vi "PicoScope6000ExampleBlockMultiUnit.vi"() -> ()   [LabVIEW 2010]
uses:
  shared/PicoBuffers.ctl
  shared/Buffer and Transfer Settings.ctl
  shared/Acquisition Settings.ctl
  PicoScope6000Lib/PicoScope6000AnalogChannelSettings.ctl
panel:
  out "Overflow":i16[](array[numeric]) format="%04b"
  in  "Trigger Settings":T1={"Trigger Enabled"=FALSE, "Trigger Source"=enum."Channel A", "Trigger Threshold (Volts)"=0.0, "Trigger Direction"=2, "Trigger Delay (samples)"=0, "Auto Trigger Time (ms)"=1000} {"Trigger Direction" items=["Rising"=2, "Falling"=3]}
  in  "Scope Index":i32
  out "Scope \"N\"":cluster{i32, sgl, "Data":dbl[]}[](graph)
  in  "Channel B Settings":T2={"Enabled"=FALSE, "Coupling"=1, "Range"=6, "Analogue Offset"=0.0, "Bandwidth"=0} {"Bandwidth" items=["Full", "20 MHz"]; "Range" items=["10 mV", "20 mV", "50 mV", "100 mV", "200 mV", "500 mV", "1 V", "2 V", "5 V", "10 V", "20 V", "50 V ", "100 V"]; "Coupling" items=["AC", "DC 1 MOhm", "DC 50 Ohm"]}
  out "Device Info":T3(array[cluster])
  out "Properties Panel":T4(array[cluster]) {"Max Total Capture Time Available (sec)" format="%.3p"; "Sample Frequency" format="%.3p"; "Sample Internal" format="%.3p"; "Max Samples Available" format="%.3p"; "Total Capture Time (sec)" format="%.3p"}
  in  "Channel A Settings":T2={"Enabled"=TRUE, "Coupling"=1, "Range"=6, "Analogue Offset"=0.0, "Bandwidth"=0} {"Bandwidth" items=["Full", "20 MHz"]; "Range" items=["10 mV", "20 mV", "50 mV", "100 mV", "200 mV", "500 mV", "1 V", "2 V", "5 V", "10 V", "20 V", "50 V ", "100 V"]; "Coupling" items=["AC", "DC 1 MOhm", "DC 50 Ohm"]}
  in  "Acquisition Settings":T5={"preTriggerSamples"=0, "postTriggerSamples"=5000000, "timebase"=5} {"postTriggerSamples" format="%_6p"; "preTriggerSamples" format="%_6p"}
  in  "Buffer and Transfer Settings":T6={"startIndex"=0, "Samples"=5000000, "Down Sample Ratio"=1, "Down-Sample Mode"=0} {"Down-Sample Mode" items=["RAW none"=2147483648, "None"=0, "Aggregate"=1, "Decimate"=2, "Average"=4]; "Down Sample Ratio" step=1; "Samples" format="%_6p"}
  in  "stop":bool
  in  "Apply Settings":bool
  in  "Serial Number":string[](array[string])
  in  "Use Serial Number":bool
  in  "error in (no error)":errorcluster
  # "Bit 0 = ChA"
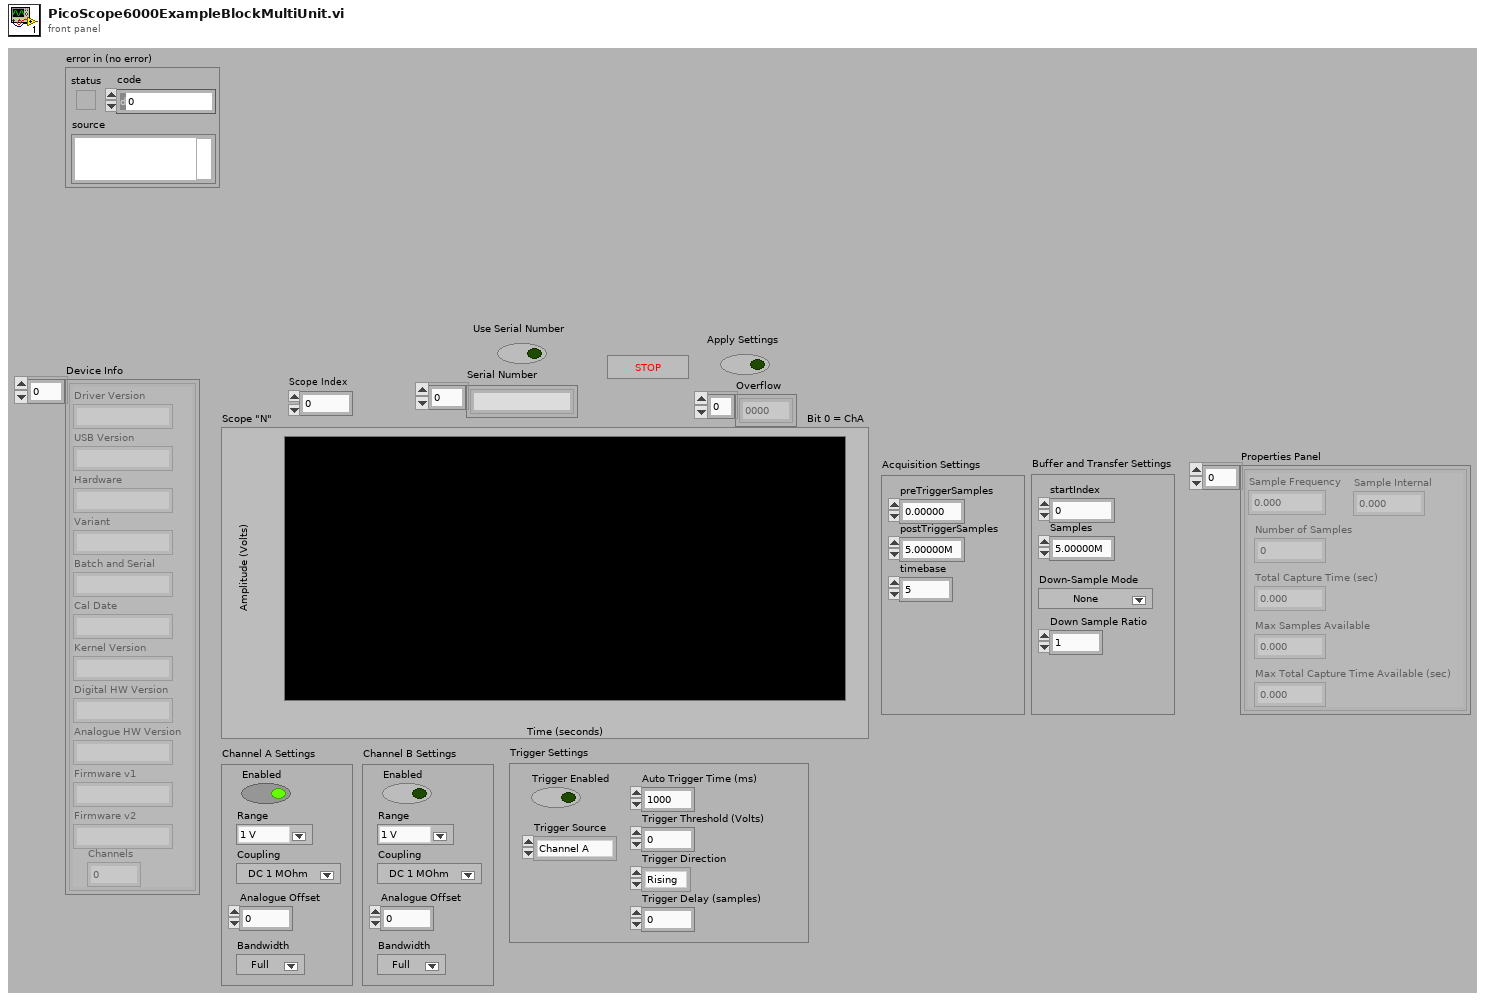
[diagram p1: front panel]
types:
  T1 = cluster{"Trigger Enabled":bool, "Trigger Source":enum32{"Channel A", "Channel B", "Channel C", "Channel D", "External", "Aux."}, "Trigger Threshold (Volts)":dbl, "Trigger Direction":u16, "Trigger Delay (samples)":u32, "Auto Trigger Time (ms)":i16}
  T2 = typedef "PicoScope6000AnalogChannelSettings.ctl" = cluster{"Enabled":bool, "Coupling":u32, "Range":u32, "Analogue Offset":sgl, "Bandwidth":u32}
  T3 = cluster{"Driver Version":string, "USB Version":string, "Hardware":string, "Variant":string, "Batch and Serial":string, "Cal Date":string, "Kernel Version":string, "Digital HW Version":string, "Analogue HW Version":string, "Firmware v1":string, "Firmware v2":string, "Channels":i16}[]
  T4 = cluster{"Sample Frequency":sgl, "Sample Internal":sgl, "maxSamples":u32, "Number of Samples":u32, "Total Capture Time (sec) ":sgl, "Max Total Capture Time Available (sec)":sgl}[]
  T5 = typedef "Acquisition Settings.ctl" = cluster{"preTriggerSamples":u64, "postTriggerSamples":u64, "timebase":u32}
  T6 = typedef "Buffer and Transfer Settings.ctl" = cluster{"startIndex":u64, "Samples":u64, "Down Sample Ratio":u64, "Down-Sample Mode":u32}
  T7 = typedef "PicoBuffers.ctl" = cluster{"Max Buffer Pointers":u64[][][], "Min Buffer Pointers":u64[][][], "StreamingDataInfo":cluster{"Channel":u32, "Down-Sample Mode":u32, "PICO_DATA_TYPE":enum32{"PICO_INT8_T", "PICO_INT16_T", "PICO_INT32_T", "PICO_UINT32_T", "PICO_INT64_T", ""}, "Samples":i32, "bufferIndex":u64, "startIndex":i32, "overflow":i16}[][]}
  T8 = cluster{"Driver Version":string, "USB Version":string, "Hardware":string, "Variant":string, "Batch and Serial":string, "Cal Date":string, "Kernel Version":string, "Digital HW Version":string, "Analogue HW Version":string, "Firmware v1":string, "Firmware v2":string, "Channels":i16}
  T9 = cluster{"Sample Frequency":sgl, "Sample Internal":sgl, "maxSamples":u32, "Number of Samples":u32, "Total Capture Time (sec) ":sgl, "Max Total Capture Time Available (sec)":sgl}
  T10 = cluster{"Channel A Buffer":i16[], "Channel B Buffer":i16[], "Channel C Buffer":i16[], "Channel D Buffer":i16[], "Channel E Buffer":i16[], "Channel F Buffer":i16[], "Channel G Buffer":i16[], "Channel H Buffer":i16[], "Port 0 Buffer":i16[], "Port 1 Buffer":i16[]}[]
  T11 = cluster{"Channel A Buffer":i16[], "Channel B Buffer":i16[], "Channel C Buffer":i16[], "Channel D Buffer":i16[], "Channel E Buffer":i16[], "Channel F Buffer":i16[], "Channel G Buffer":i16[], "Channel H Buffer":i16[], "Port 0 Buffer":i16[], "Port 1 Buffer":i16[]}
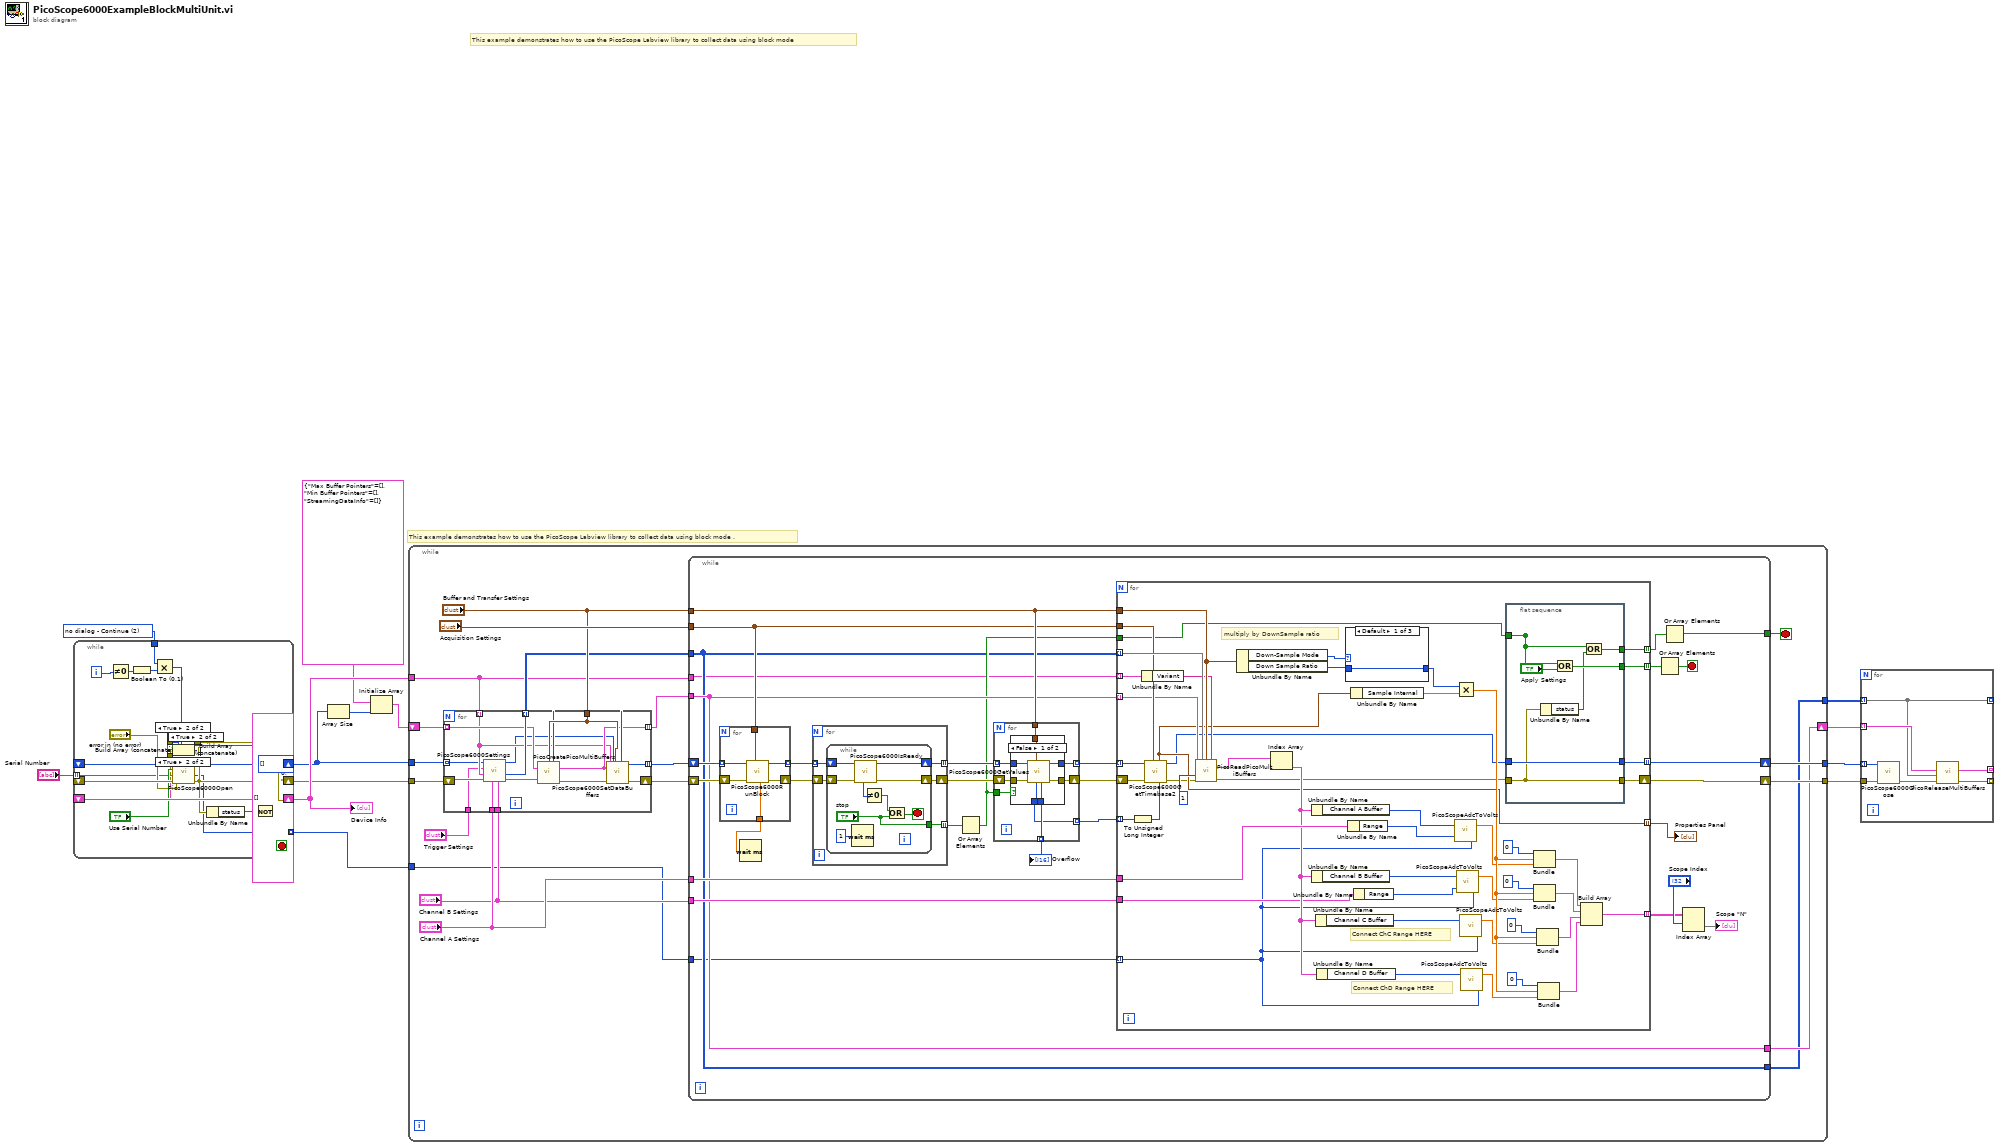
[diagram p0: block diagram]
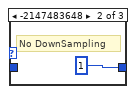
[diagram p5: hidden frame]
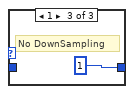
[diagram p6: hidden frame]
diagram:
  w16 = u16 2 items=["Dialog On Error", "no dialog - CloseUnit and Stop", "no dialog - Continue", "no dialog - Stop"] ("Mode")
  # "This example demonstrates how to use the PicoScope Labview library to collect data using block mode ."
  # "This example demonstrates how to use the PicoScope Labview library to collect data using block mode"
  n1 = while {
    tunnel: w16 -> [w30]
    tunnel: "Serial Number" -> [w27] mode=indexing
    tunnel: [w26] -> w8 mode=indexing
    shift-right: [w21] -> w14
    shift-left: errorcluster {"status"=FALSE, "code"=0, "source"=""} ("error out") -> [w22]
    shift-right: [w19] -> w10
    shift-left: i16[] [] ("Array") -> [w20]
    shift-right: [w17] -> w15
    shift-left: T3 [] ("Array") -> [w18]
    i -> [w31]
    stop <- w23 stop-if-true
    n2 = Not Equal To 0?(x=w31) -> (x != 0?=w33:bool)
    n3 = Boolean To (0,1)(Boolean=w33) -> (0, 1=w32:i16)
    n4 = Multiply(x=w30, y=w32) -> (x*y=w29:u16)
    n5 = call "PicoScope6000Open.vi"("Mode"=w29, "error in (no error)"="error in (no error)", "Serial Number"=w27, "Use Serial Number"="Use Serial Number") -> ("error out"=w28:errorcluster, "Max Adc value"=w26:i16, "handle"=w25:i16, "Device Info"=w34:T8)  [unwired: 3 in, 1 out]
    n6 = Unbundle By Name(w28) -> ("status"=w23:bool)
    n7 = Not(x=w23) -> (.not. x?=w24:bool)
    n8 = case shown="True" w24 {
      tunnel: w18 -> [w37 w39]
      tunnel: w34 -> [_ w38]
      tunnel: [w37 w40] -> w17
      frame False {
      }
      frame True {
        n9 = Build Array (concatenate)(w39, w38) -> (w40:T3)
      }
    }
    n10 = case shown="True" w24 {
      tunnel: w20 -> [w41 w43]
      tunnel: w25 -> [_ w42]
      tunnel: [w41 w44] -> w19
      frame False {
      }
      frame True {
        n11 = Build Array (concatenate)(w43, w42) -> (w44:i16[])
      }
    }
    n12 = case shown="True" w24 {
      tunnel: w22 -> [w45 _]
      tunnel: w28 -> [_ w46]
      tunnel: [w45 w46] -> w21
      frame False {
      }
      frame True {
      }
    }
  }
  "Device Info" <- w15
  n13 = Array Size(array=w10) -> (size(s)=w12:i32)
  n14 = Initialize Array(T7 {"Max Buffer Pointers"=[], "Min Buffer Pointers"=[], "StreamingDataInfo"=[]} ("Data Pointers"), w12) -> (w9:T7[])
  n15 = while {
    tunnel: w14 -> [w50]
    tunnel: [w49] -> w5
    tunnel: w15 -> [w55]
    tunnel: w10 -> [w51]
    tunnel: [w64] -> w7
    tunnel: [w62] -> w4
    shift-right: [w52] -> w6
    shift-left: w9 -> [w53]
    tunnel: w8 -> [w48]
    stop <- w63 stop-if-true
    n16 = for {
      tunnel: [w79] -> w60 mode=indexing
      tunnel: "Channel A Settings" -> [w77]
      tunnel: "Buffer and Transfer Settings" -> [w76]
      tunnel: [w75] -> w57 mode=indexing
      tunnel: w55 -> [w71] mode=indexing
      tunnel: "Channel B Settings" -> [w73]
      tunnel: w51 -> [w69] mode=indexing
      shift-right: [w80] -> w61
      shift-left: w50 -> [w70]
      tunnel: w53 -> [w72] mode=indexing
      tunnel: [w74] -> w56 mode=indexing
      tunnel: "Trigger Settings" -> [w66]
      n17 = call "PicoScope6000Settings.vi"("Channel B Settings"=w73, "Channel A Settings"=w77, "error in"=w70, "Device Info"=w71, "Trigger Settings"=w66, "handle in"=w69) -> ("error out"=w68:errorcluster, "Enabled array"=w75:i16[], "handle out"=w67:i16)  [unwired: 3 in]
      n18 = call "PicoCreatePicoMultiBuffers.vi"("Buffer and Transfer Settings"=w76, "enabled array"=w75, "Data Pointers In"=w72, "error in (no error)"=w68) -> ("Data Pointers"=w74:T7, "error out"=w78:errorcluster)  [unwired: 10 in]
      n19 = call "PicoScope6000SetDataBuffers.vi"("enabled array"=w75, "Buffer and Transfer Settings"=w76, "error in (no error)"=w78, "Device Info"=w71, "Data Pointers In"=w74, "handle in"=w67) -> ("error out"=w80:errorcluster, "handle out"=w79:i16)  [unwired: 4 in]
    }
    n20 = while {
      tunnel: w56 -> [w95]
      tunnel: "Buffer and Transfer Settings" -> [w105]
      tunnel: w57 -> [w85]
      tunnel: "Channel A Settings" -> [w111]
      tunnel: "Acquisition Settings" -> [w97]
      tunnel: w55 -> [w84]
      tunnel: [w89] -> w63
      shift-right: [w110] -> w64
      shift-left: w61 -> [w103]
      shift-right: [w109] -> w62
      shift-left: w60 -> [w104]
      tunnel: "Channel B Settings" -> [w96]
      tunnel: [w95] -> w52
      tunnel: [w85] -> w49
      tunnel: w48 -> [w83]
      stop <- w90 stop-if-true
      n21 = for {
        tunnel: [w203] -> w100
        tunnel: w97 -> [w202]
        shift-right: [w205] -> w102
        shift-left: w103 -> [w206]
        tunnel: w104 -> [w207] mode=indexing
        tunnel: [w204] -> w101 mode=indexing
        n22 = call "PicoScope6000RunBlock.vi"("Acquisition Settings"=w202, "error in (no error)"=w206, "handle in"=w207) -> ("error out"=w205:errorcluster, "handle out"=w204:i16, "timeIndisposedMs"=w203:dbl)  [unwired: 5 in, 1 out]
      }
      n23 = Wait (ms)(milliseconds to wait=w100) -> ()  [unwired: 1 out]
      n24 = for {
        tunnel: [w192] -> w108 mode=indexing
        tunnel: [w190] -> w94 mode=indexing
        tunnel: w101 -> [w188] mode=indexing
        shift-right: [w191] -> w107
        shift-left: w102 -> [w189]
        n25 = while {
          shift-right: [w194] -> w191
          shift-left: w189 -> [w198]
          shift-right: [w195] -> w192
          shift-left: w188 -> [w197]
          tunnel: ["stop"] -> w190
          stop <- w200 stop-if-true
          n26 = Wait (ms)(milliseconds to wait=u32 1) -> ()  [unwired: 1 out]
          n27 = call "PicoScope6000IsReady.vi"("error in (no error)"=w198, "handle in"=w197) -> ("error out"=w194:errorcluster, "handle out"=w195:i16, "ready"=w193:i16)  [unwired: 7 in]
          n28 = Not Equal To 0?(x=w193) -> (x != 0?=w201:bool)
          n29 = Or(x=w201, y="stop") -> (x .or. y?=w200:bool)
        }
      }
      n30 = Or Array Elements(Boolean array=w94) -> (logical OR=w93:bool)
      n31 = for {
        tunnel: w108 -> [w178] mode=indexing
        tunnel: [w176] -> w81 mode=indexing
        tunnel: [w175] -> w106 mode=indexing
        tunnel: w105 -> [w174]
        tunnel: [w172] -> w98 mode=indexing
        tunnel: w93 -> [w171]
        shift-right: [w173] -> w99
        shift-left: w107 -> [w177]
        n32 = case shown="False" w171 {
          tunnel: w177 -> [w184 w186]
          tunnel: w178 -> [w183 w187]
          tunnel: [w182 w187] -> w172
          tunnel: [w185 w186] -> w173
          tunnel: w174 -> [w181 _]
          tunnel: [w180 _] -> w176
          tunnel: [w179 _] -> w175
          frame False {
            n33 = call "PicoScope6000GetValues.vi"("Buffer and Transfer Settings"=w181, "error in (no error)"=w184, "handle in"=w183) -> ("error out"=w185:errorcluster, "handle out"=w182:i16, "overflow"=w180:i16, "noOfSamples"=w179:u64)  [unwired: 5 in]
          }
          frame True {
          }
        }
      }
      "Overflow" <- w81
      n34 = for {
        tunnel: w85 -> [w155] mode=indexing
        tunnel: w111 -> [w154]
        tunnel: [w131] -> w92 mode=indexing
        tunnel: [w130] -> w109 mode=indexing
        tunnel: w106 -> [w129] mode=indexing
        tunnel: w105 -> [w128]
        tunnel: w98 -> [w115] mode=indexing
        tunnel: w97 -> [w126]
        tunnel: w96 -> [w124]
        tunnel: w95 -> [w123] mode=indexing
        shift-right: [w133] -> w110
        shift-left: w99 -> [w116]
        tunnel: [w121] -> w86 mode=indexing
        tunnel: w93 -> [w122]
        tunnel: [w132] -> w91 mode=indexing
        tunnel: w84 -> [w120] mode=indexing
        tunnel: w83 -> [w118] mode=indexing
        tunnel: [w117] -> w82 mode=indexing
        # "Connect ChD Range HERE"
        # "Connect ChC Range HERE"
        # "multiply by DownSample ratio"
        n35 = To Unsigned Long Integer(number=w129) -> (unsigned 32bit integer=w127:u32)
        n36 = Unbundle By Name(w120) -> ("Variant"=w119:string)
        n37 = call "PicoScope6000GetTimebase2.vi"("Number of Samples"=w127, "Acquisition Settings"=w126, "error in (no error)"=w116, "handle in"=w115) -> ("error out"=w114:errorcluster, "handle out"=w113:i16, "Properties Panel"=w117:T9)  [unwired: 5 in]
        n38 = call "PicoReadPicoMultiBuffers.vi"("enabled array"=w155, "Buffer and Transfer Settings"=w128, "Variant"=w119, "Data Pointers"=w123, "No of Buffers"=1, "error in (no error)"=w114) -> ("MultiBuffers (Max or non-aggregated)"=w160:T10, "error out"=w112:errorcluster)  [unwired: 7 in, 1 out]
        n39 = Unbundle By Name(w128) -> ("Down-Sample Mode"=w158:u32, "Down Sample Ratio"=w159:u64)
        n40 = Index Array(array=w160) -> (element=w134:T11)  [unwired: 1 in]
        n41 = Unbundle By Name(w134) -> ("Channel A Buffer"=w143:i16[])
        n42 = Unbundle By Name(w134) -> ("Channel B Buffer"=w148:i16[])
        n43 = Unbundle By Name(w134) -> ("Channel C Buffer"=w141:i16[])
        n44 = Unbundle By Name(w134) -> ("Channel D Buffer"=w137:i16[])
        n45 = case shown="Default" w158 {
          tunnel: [w168 u64 1 ("Down Sample Ratio") u64 1 ("Down Sample Ratio")] -> w156
          tunnel: w159 -> [w168 _ _]
          frame Default {
          }
          frame -2147483648 {
            # "No DownSampling"
          }
          frame 1 {
            # "No DownSampling"
          }
        }
        n46 = Unbundle By Name(w154) -> ("Range"=w150:u32)
        n47 = Unbundle By Name(w117) -> ("Sample Internal"=w153:sgl)
        n48 = Unbundle By Name(w124) -> ("Range"=w125:u32)
        n49 = call "PicoScopeAdcToVolts.vi"("Max_adc"=w118, "Range Index"=w150, "Data"=w143) -> ("Data"=w144:dbl[])
        n50 = Multiply(x=w156, y=w153) -> (x*y=w157:sgl)
        n51 = call "PicoScopeAdcToVolts.vi"("Max_adc"=w118, "Range Index"=w125, "Data"=w148) -> ("Data"=w147:dbl[])
        n52 = call "PicoScopeAdcToVolts.vi"("Max_adc"=w118, "Data"=w141) -> ("Data"=w140:dbl[])  [unwired: 1 in]
        n53 = call "PicoScopeAdcToVolts.vi"("Max_adc"=w118, "Data"=w137) -> ("Data"=w136:dbl[])  [unwired: 1 in]
        n54 = flat-sequence {
          tunnel: [w167] -> w131
          tunnel: [w162] -> _
          tunnel: [w164] -> w132
          tunnel: w113 -> [w163]
          tunnel: [w163] -> w130
          tunnel: [w161] -> w133
          tunnel: w122 -> [w162]
          tunnel: w112 -> [w161]
          frame #0 {
            n55 = Unbundle By Name(w161) -> ("status"=w165:bool)
            n56 = Or(x=w162, y="Apply Settings") -> (x .or. y?=w167:bool)
            n57 = Or(x=w162, y=w165) -> (x .or. y?=w164:bool)
          }
        }
        n58 = Bundle(0, w157, "Data"=w144) -> (w146:cluster{i32, sgl, "Data":dbl[]})  [unwired: 1 in]
        n59 = Bundle(0, w157, "Data"=w147) -> (w145:cluster{i32, sgl, "Data":dbl[]})  [unwired: 1 in]
        n60 = Bundle(0, w157, "Data"=w140) -> (w139:cluster{i32, sgl, "Data":dbl[]})  [unwired: 1 in]
        n61 = Bundle(0, w157, "Data"=w136) -> (w135:cluster{i32, sgl, "Data":dbl[]})  [unwired: 1 in]
        n62 = Build Array(w146, w145, w139, w135) -> (w121:cluster{i32, sgl, "Data":dbl[]}[])
      }
      "Properties Panel" <- w82
      n63 = Or Array Elements(Boolean array=w92) -> (logical OR=w90:bool)
      n64 = Or Array Elements(Boolean array=w91) -> (logical OR=w89:bool)
      n65 = Index Array(array=w86, index (row)="Scope Index") -> (element=→"Scope \"N\"":cluster{i32, sgl, "Data":dbl[]}[])  [unwired: 1 in]
    }
  }
  n66 = for {
    tunnel: w5 -> [w211] mode=indexing
    tunnel: w6 -> [w214] mode=indexing
    tunnel: w7 -> [w210]
    tunnel: [w213] -> _ mode=indexing
    tunnel: [w212] -> _ mode=indexing
    tunnel: [w211] -> _ mode=indexing
    tunnel: w4 -> [w208] mode=indexing
    n67 = call "PicoScope6000Close.vi"("error in (no error)"=w210, "handle"=w208) -> ("error out"=w209:errorcluster)  [unwired: 8 in, 1 out]
    n68 = call "PicoReleaseMultiBuffers.vi"("error in (no error)"=w209, "Enabled array"=w211, "Data Pointers"=w214) -> ("error out"=w213:errorcluster, "Data Pointers Out"=w212:T7)  [unwired: 7 in]
  }
